vi "TEST - List Directory.vi"(8 "error in (no error)":errorcluster) -> (0 "error out":errorcluster, 2 "pass":bool)   [LabVIEW 2020]
uses:
  <userlib>/_OpenG.lib/error/error.llb/openg_error.lvlib
  source/library/Build Path/Build Path - File Names Array.vi
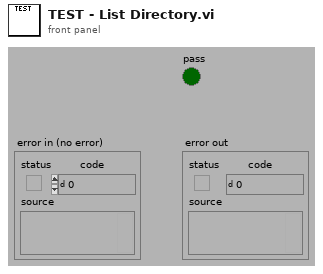
[diagram p1: front panel]
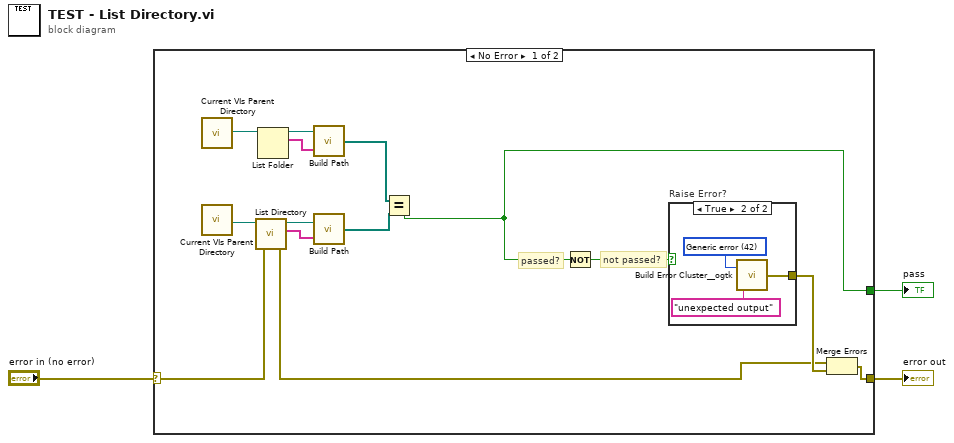
[diagram p0: block diagram]
diagram:
  n1 = case shown="No Error" "error in (no error)" {
    selector: "error in (no error)" -> [w13 w21]
    tunnel: [w4 _] -> w3
    tunnel: [w17 w21] -> w1
    frame No Error {
      # "not passed?"
      # "passed?"
      n2 = call "Current VIs Parent Directory.vi"() -> ("Parent Directory (+ Relative)"=w12:path)  [unwired: 5 in]
      n3 = call "Current VIs Parent Directory.vi"() -> ("Parent Directory (+ Relative)"=w11:path)  [unwired: 5 in]
      n4 = call "List Directory.vi"("error in (no error)"=w13, "directory path"=w11) -> ("error out"=w14:errorcluster, "file names"=w7:string[], "dup directory path"=w8:path)  [unwired: 2 in, 1 out]
      n5 = List Folder(path=w12) -> (path out=w10:path, filenames=w9:string[])  [unwired: 3 in, 2 out]
      n6 = call-poly "Build Path.vi"("name or relative path"=w9, "base path"=w10) -> ("appended path"=w5:path[])
      n7 = call-poly "Build Path.vi"("name or relative path"=w7, "base path"=w8) -> ("appended path"=w6:path[])
      n8 = Equal?(x=w5, y=w6) -> (x = y?=w4:bool)
      n9 = Not(x=w4) -> (.not. x?=w15:bool)
      n10 = case "Raise Error?" shown="True" w15 {
        tunnel: [_ w18] -> w16
        frame False {
        }
        frame True {
          w19 = 42 items=["No error", "Argument error", "Memory is full", "Out of zone", "End of file", "File already open", "Generic file I/O error", "File not found", "File permission error", "Disk is full", "Duplicate path", "Too many files open", "System feature not enabled", "Resource file not found", "Cannot add resource", "Resource not found", "Image not found", "Image memory error", "Pen does not exist", "Config type invalid", "Config token not found", "Config parse error", "Config memory error", "Bad external code format", "Bad external code offset", "External code not present", "Null window", "Destroy window error", "Null menu", "Print aborted", "Bad print record", "Print driver error", "Windows error during printing", "Memory error during printing", "Print dialog error", "Generic print error", "Invalid device refnum", "Device not found", "Device parameter error", "Device unit error", "Cannot open device", "Device call aborted", "Generic error", "Cancelled by user", "Object ID too low", "Object ID too high", "Object not in heap", "Unknown heap", "Unknown object (invalid DefProc)", "Unknown object (DefProc not in table)", "Message out of range", "Invalid (null) method", "Unknown message", "Manager call not supported", "Bad address", "Network operation in progress", "Network operation timed out", "Connection is busy", "Network attribute not supported", "Network error", "Address in use", "System out of memory", "Connection aborted", "Connection refused", "Not connected", "Already connected", "Connection closed", "Initialization error (interapplication manager)", "Bad occurrence", "Wait on unbound occurrence handler", "Occurrence queue overflow", "Datalog type conflict", "Unused", "Unrecognized type (interapplication manager)", "Memory corrupt", "Failed to make temporary DLL", "Old CIN version", "Drag socket not found", "Failed to load drop-object", "Failed to register OLE object", "Failed to release OLE object", "Format specifier type mismatch", "Unknown format specifier", "Too few format specifiers", "Too many format specifiers", "Scan failed", "Newer CIN version", "Error converting to variant", "Runtime menu error", "Password tampered", "Variant attribute not found", "Incompatible variant data type", "Event data is not available", "Event Store is not present", "Occurrence is not found", "Event Queue is not created", "Event info is not available", "Refnum passed is NULL", "Error retrieving Class GUID", "Error retrieving CoClass GUID", "Error retrieving TypeLib GUID.", "Bad built application magic bytes.", "Specific driver is different from the specific driver associated with the Logical Name.", "There is no session opened to the class driver.", "Max Error", "MAX - Error with config objects", "MAX - Error loading configuration", "MAX - Group not supported"]
          n11 = call <userlib>:"Build Error Cluster__ogtk.vi"("String to Prepend to source (\"\")"="unexpected output" ("String to Prepend to source (\"\")"), "code"=w19) -> ("error out"=w18:errorcluster)
        }
      }
      n12 = Merge Errors(w14, w16) -> (w17:errorcluster)
    }
    frame Error {
    }
  }
  "pass" <- w3
  "error out" <- w1
